vi "Stage and Sensor.vi"() -> ()   [LabVIEW 2025]
uses:
  \\chem-fs-prd-01\cyran_research/Users/Erykah F/Vertical Stage + Sensor/ThorLabs.MotionControl.KCube.PositionAlignerCLI.dll
  Vertical Stage + Sensor/ThorLabs.MotionControl.KCube.PositionAlignerCLI.dll
  Vertical Stage + Sensor/libximc.lvlib
  \\chem-fs-prd-01\cyran_research/Users/Erykah F/Vertical Stage + Sensor/Thorlabs.MotionControl.Controls.dll
  Vertical Stage + Sensor/Thorlabs.MotionControl.Controls.dll
panel:
  out "Y diff":dbl
  out "X diff":dbl
  out "Sum":dbl
  in  "KCubePositionAlignerControl":refnum<k24>(container)
  in  "Tab Control":T1(tab)
  in  "Controller 3":u16(ring) items=["xi-com:\\\\.\\COM4", "xi-com:\\\\.\\COM5", "xi-com:\\\\.\\COM6"]
  in  "Controller 2":u16(ring) items=["xi-com:\\\\.\\COM4", "xi-com:\\\\.\\COM5", "xi-com:\\\\.\\COM6"]
  in  "Controller 1":u16(ring) items=["xi-com:\\\\.\\COM4", "xi-com:\\\\.\\COM5", "xi-com:\\\\.\\COM6"]
  out "s/n 1":u32
  out "s/n 3":u32
  out "s/n 2":u32
  in  "KCube Serial  Number":string="69254064"
  in  "Move To Destination":bool
  in  "Move Relative":bool
  in  "Shift 1":i32
  in  "Shift 2":i32
  in  "Shift 3":i32
  in  "Destination 3":i32
  in  "Destination 2":i32
  in  "Destination 1":i32
  in  "Loop?":bool caption="Loop Shift?"
  in  "Shift Amount (Steps)":i32=1
  in  "Wait Time (s)":dbl=1.0
  in  "Exit":bool
  out "Cursor 3":dbl format="%#.2f"
  out "Cursor 2":dbl format="%#.2f"
  out "Cursor 1":dbl format="%#.2f"
  # "Position Status"
  # "\\_(-_ -)_/"
  # "Controller IDs"
  # "Serial Numbers"
  # "Disabled because we don't usually use this function"
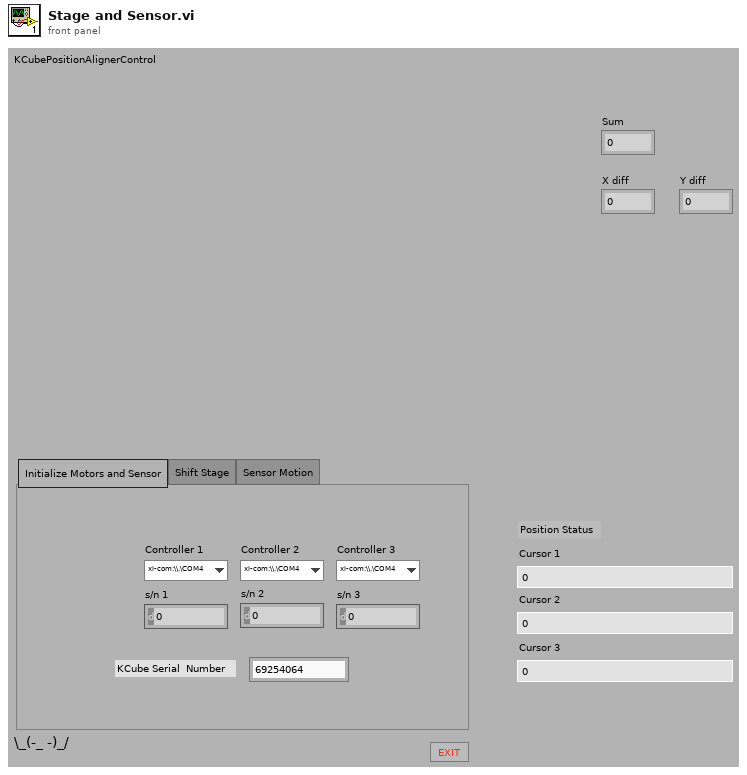
[diagram p1: front panel]
types:
  T1 = enum32{"Initialize Motors and Sensor", "Shift Stage", "Sensor Motion"}
  T2 = cluster{"Number of controllers":i32, "Controllers' names":string[], "variant":variant, "quit":bool, "IDs":i32[]}
  T3 = cluster{"KCubePositionAlignerControl":refnum<k24>, "Device":refnum<k24>, dbl, dbl, dbl, dbl}
  T4 = cluster{"MoveSts":u32, "MvCmdSts":u32, "PWRSts":u32, "EncSts":u32, "WindSts":u32, "CurPosition":i32, "uCurPosition":i32, "@dummy control@":i8, "@dummy control@":i8, "@dummy control@":i8, "@dummy control@":i8, "EncPosition":i64, "CurSpeed":i32, "uCurSpeed":i32, "Ipwr":i32, "Upwr":i32, "Iusb":i32, "Uusb":i32, "CurT":i32, "Flags":u32, "GPIOFlags":u32, "CmdBufFreeSpace":u32}
  T5 = cluster{"Shift 1":i32, "Shift 2":i32, "Shift 3":i32}
  T6 = cluster{"Destination 1":i32, "Destination 2":i32, "Destination 3":i32}
  T7 = cluster{"Shift Amount (Steps)":i32, "Shift Amount (Steps)":i32, "Shift Amount (Steps)":i32}
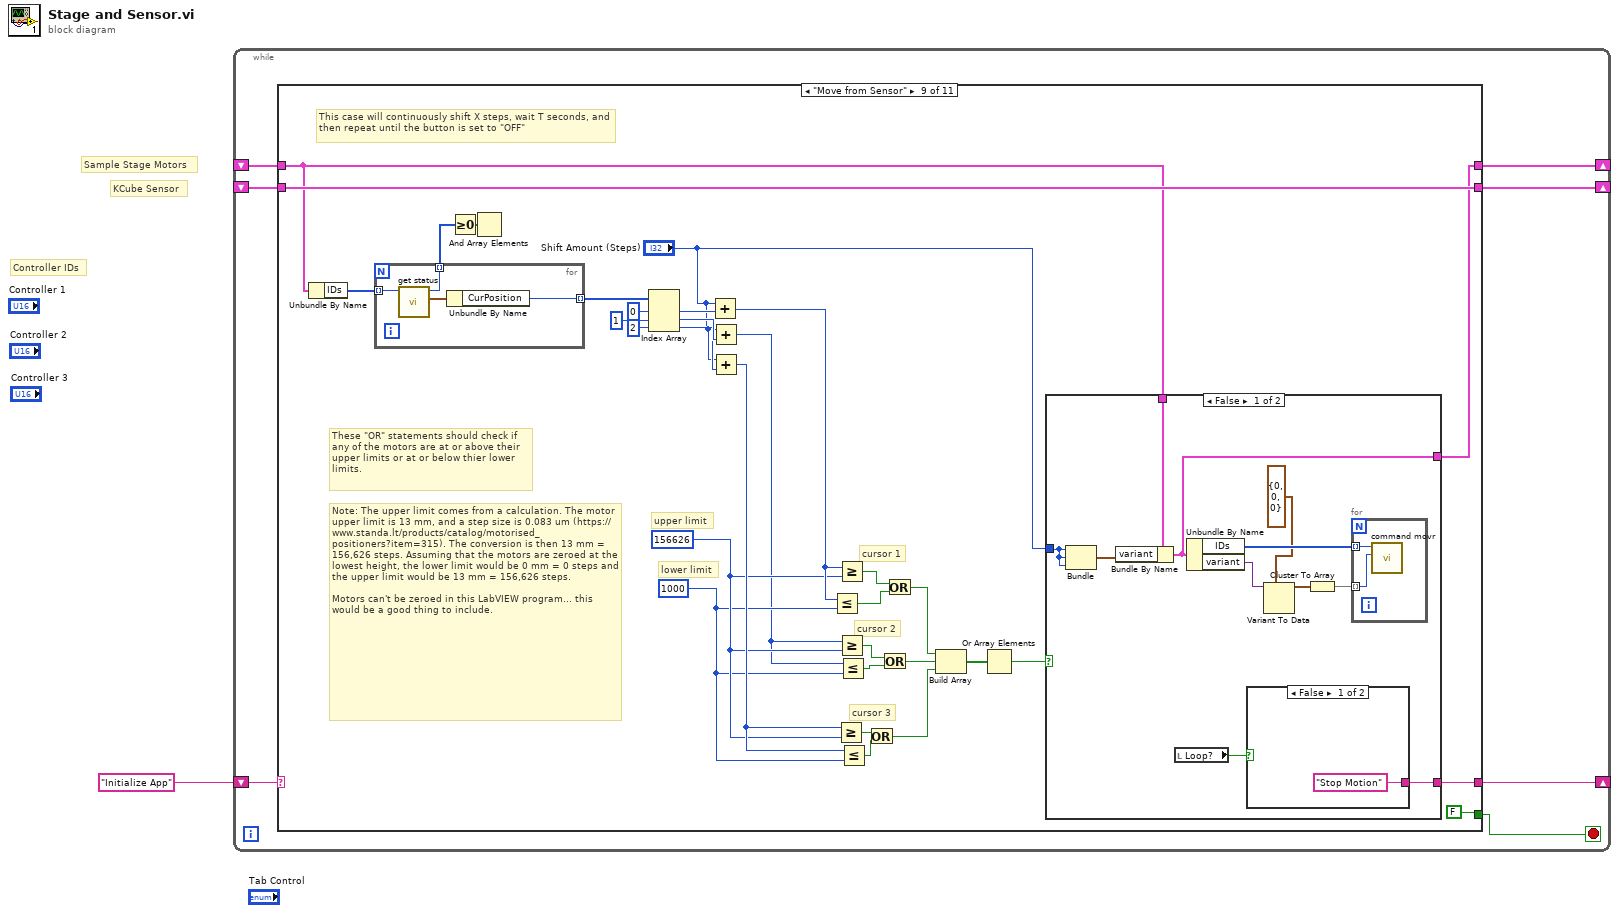
[diagram p0: block diagram]
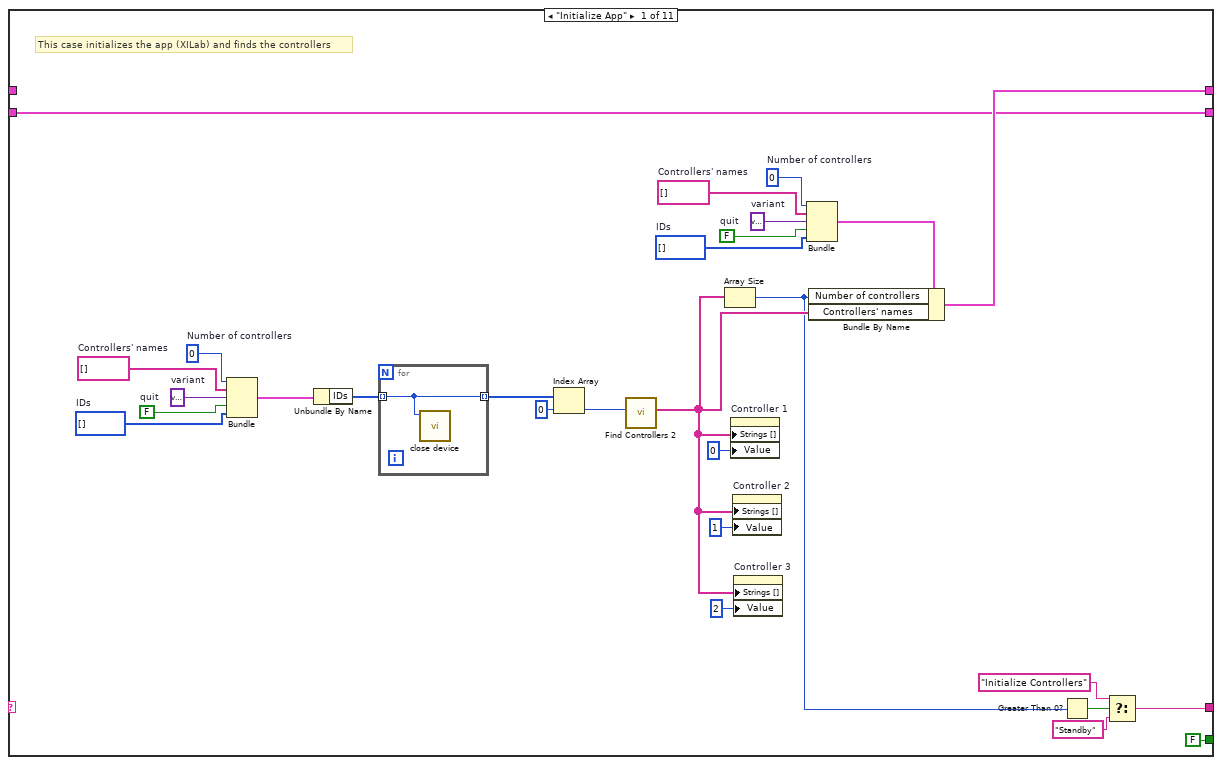
[diagram p2: hidden frame]
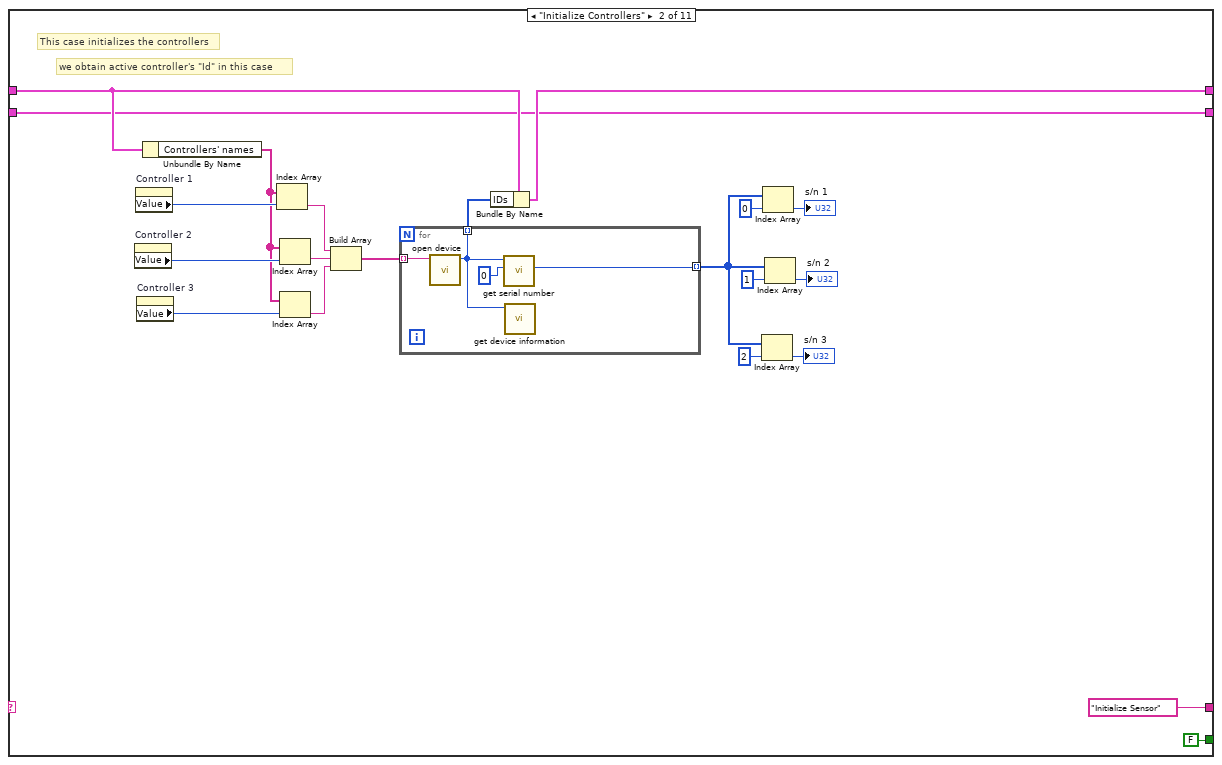
[diagram p3: hidden frame]
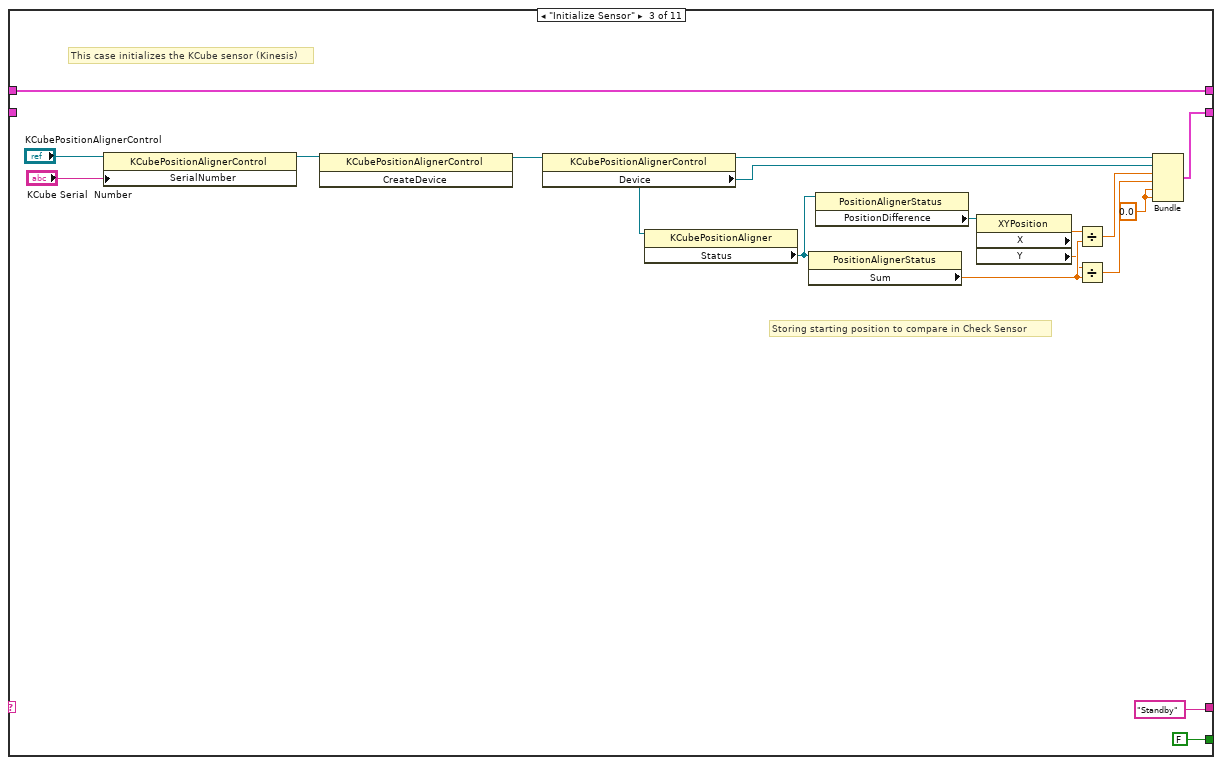
[diagram p4: hidden frame]
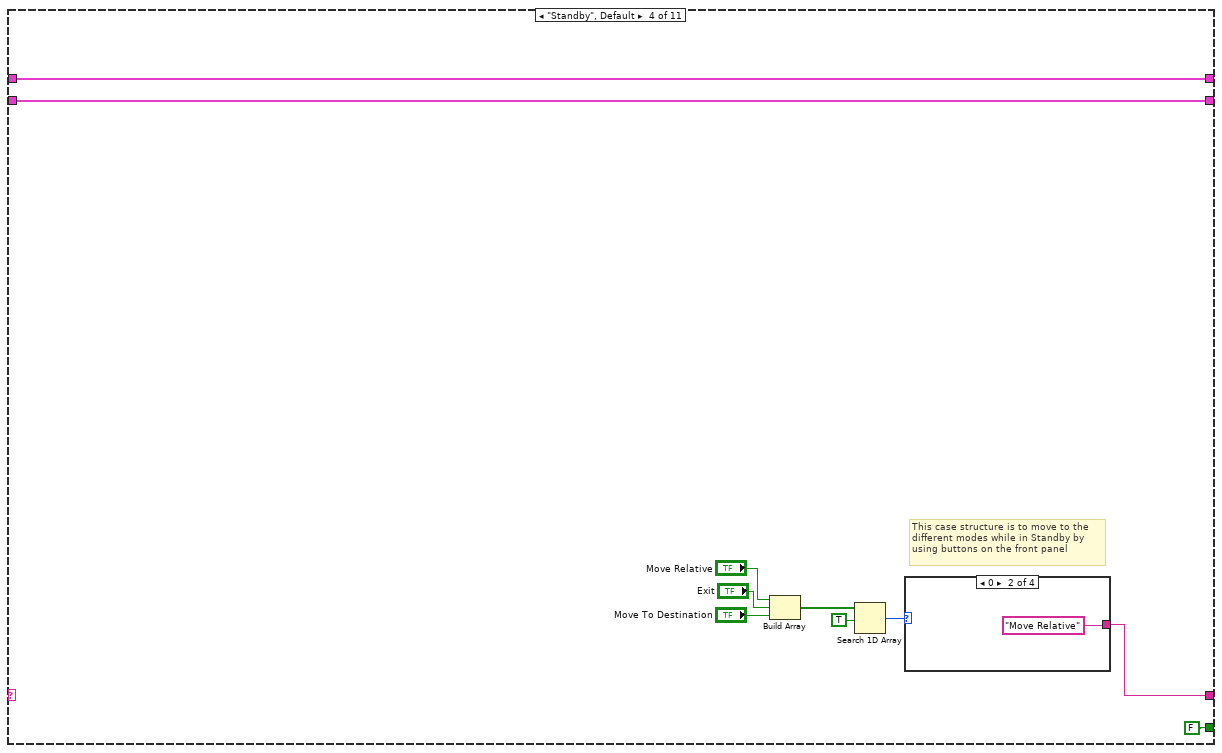
[diagram p5: hidden frame]
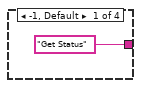
[diagram p6: hidden frame]
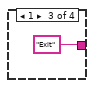
[diagram p7: hidden frame]
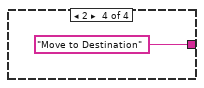
[diagram p8: hidden frame]
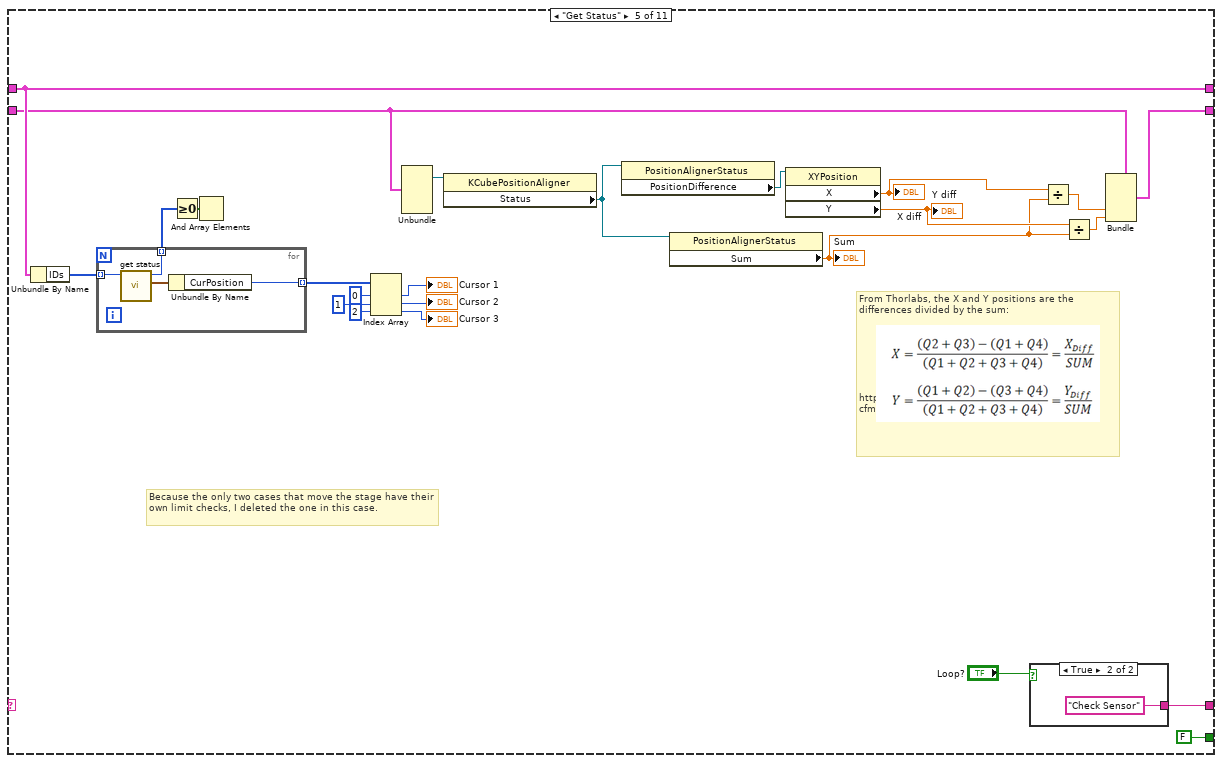
[diagram p9: hidden frame]
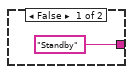
[diagram p10: hidden frame]
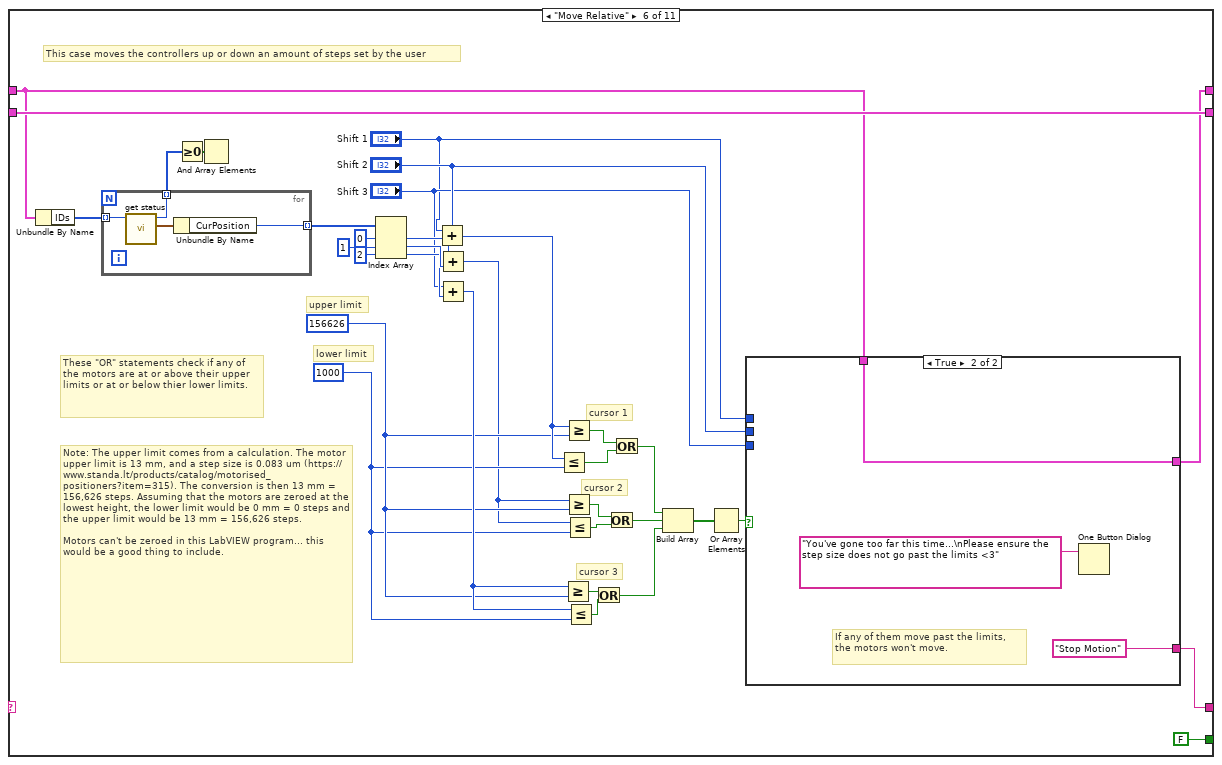
[diagram p11: hidden frame]
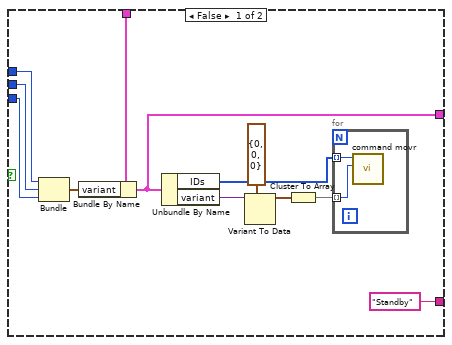
[diagram p12: hidden frame]
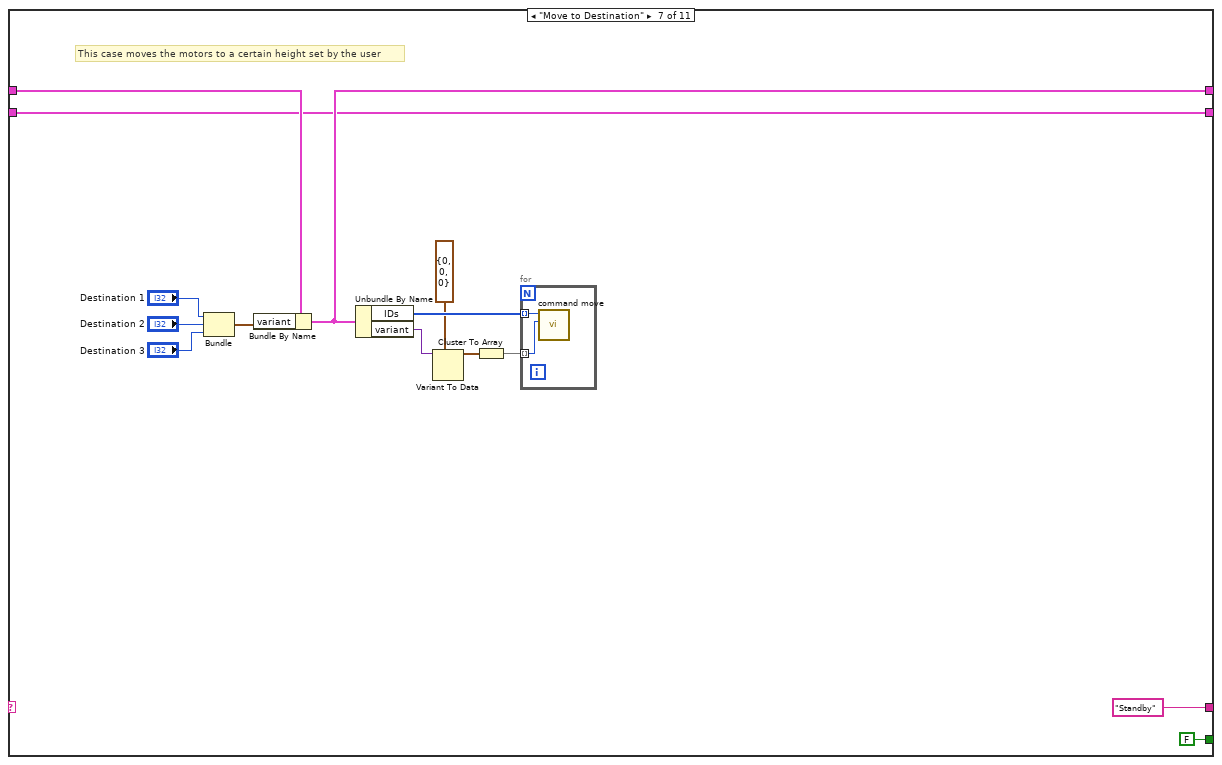
[diagram p13: hidden frame]
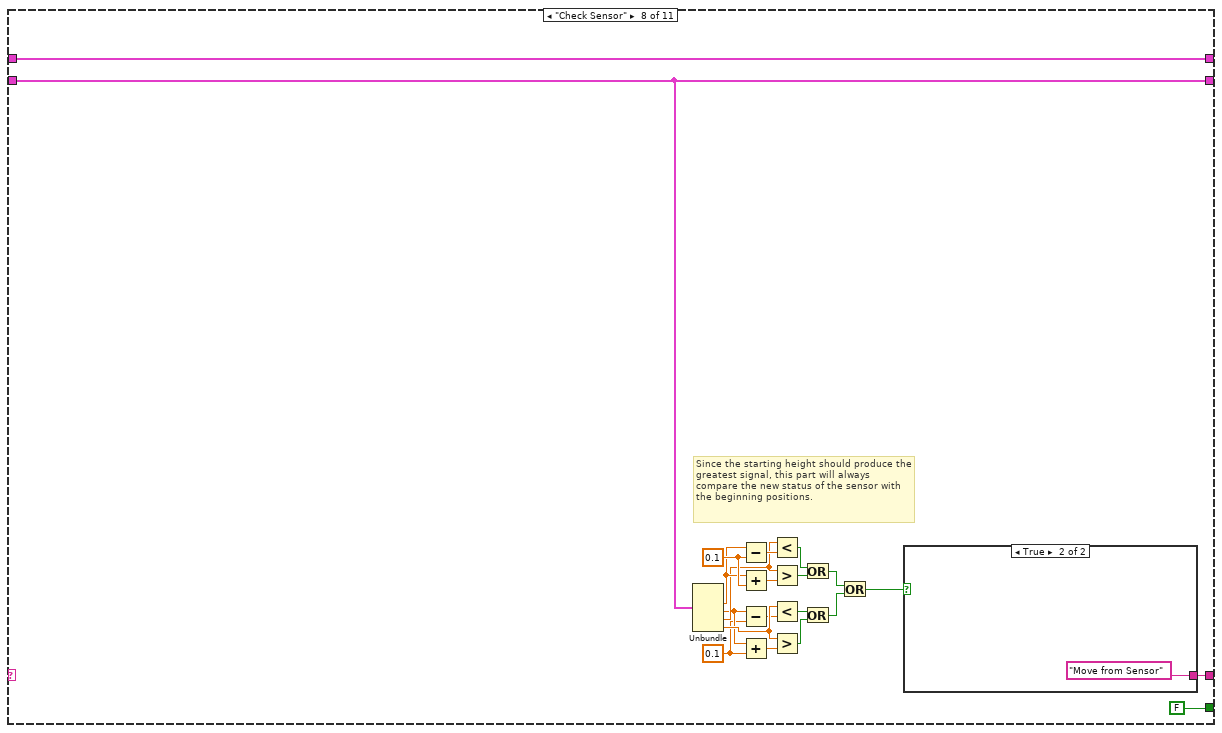
[diagram p14: hidden frame]
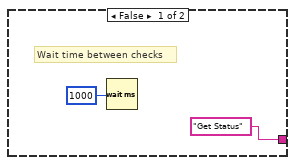
[diagram p15: hidden frame]
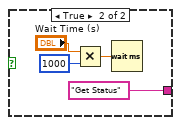
[diagram p16: hidden frame]
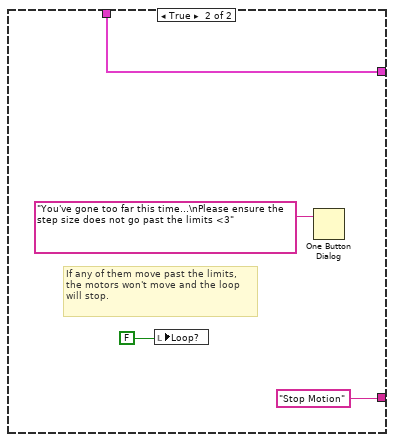
[diagram p17: hidden frame]
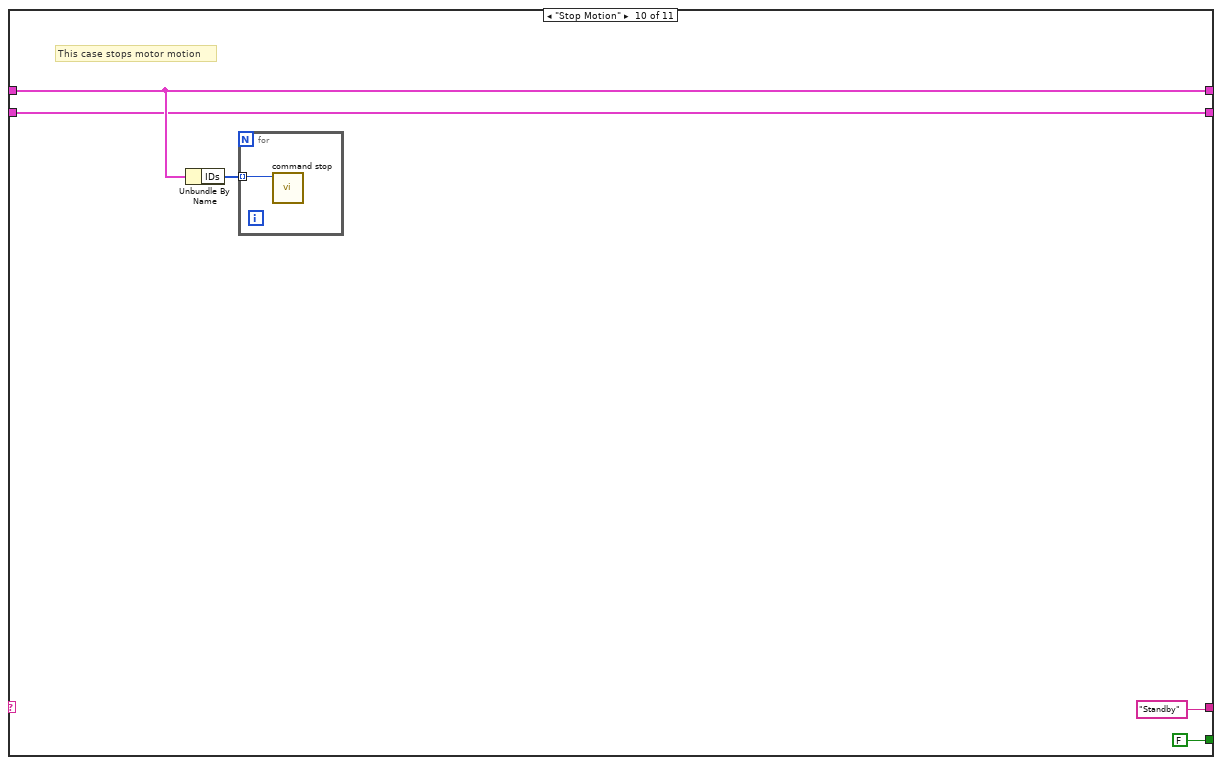
[diagram p18: hidden frame]
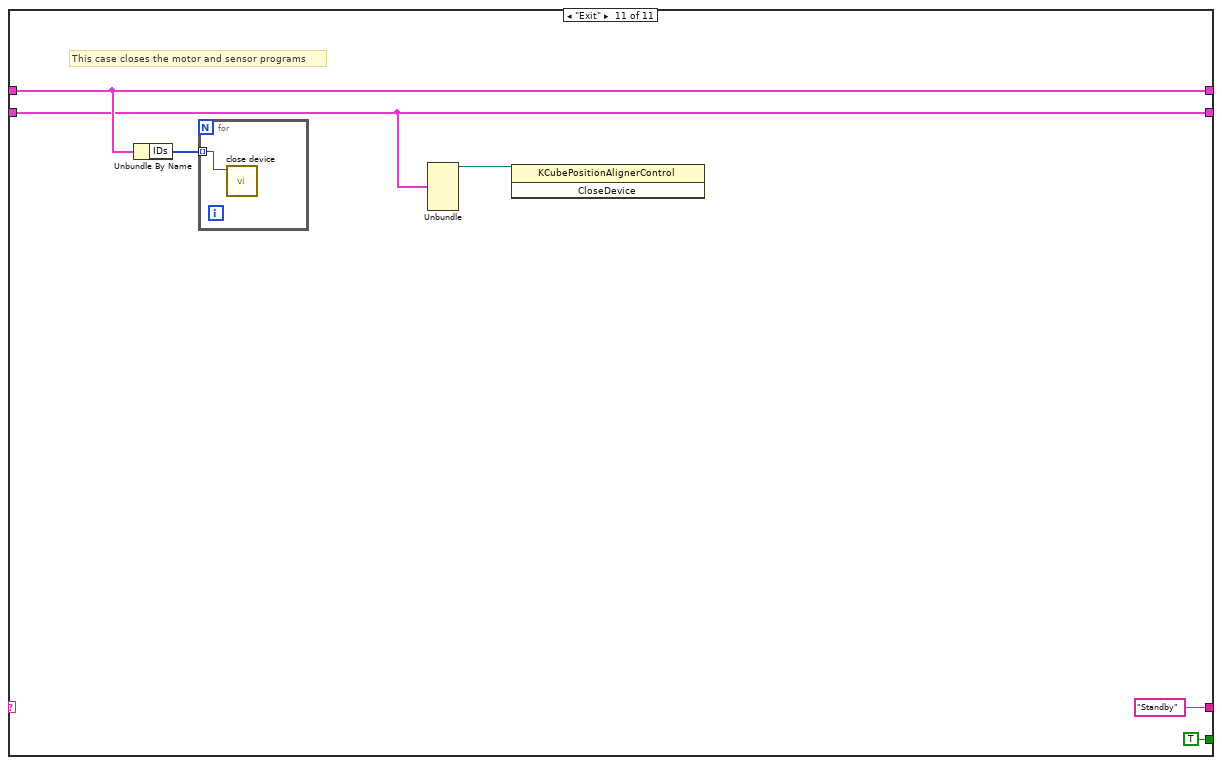
[diagram p19: hidden frame]
diagram:
  # "KCube Sensor"
  # "Sample Stage Motors"
  # "Controller IDs"
  n1 = while {
    shift-right: [w7] -> _
    shift-left: _ -> [w8]
    shift-right: [w6] -> _
    shift-left: "Initialize App" -> [w5]
    shift-right: [w3] -> _
    shift-left: _ -> [w2]
    stop <- w4 stop-if-true
    n2 = case shown="\"Move from Sensor\"" w5 {
      tunnel: [w30 w48 w79 w90 w111 w126 w182 w216 w221 w279 w287] -> w7
      tunnel: w8 -> [_ w49 w79 w90 w111 w127 w184 w216 w222 w279 w287]
      tunnel: [w11 "Initialize Sensor" "Standby" w84 w96 w139 "Standby" w214 w251 "Standby" "Standby"] -> w6
      tunnel: [FALSE ("quit") FALSE ("quit") FALSE FALSE ("quit") FALSE ("quit") FALSE ("quit") FALSE ("quit") FALSE FALSE FALSE TRUE ("quit")] -> w4
      tunnel: [w9 w38 w73 w82 w104 w158 w180 w213 w249 w278 w284] -> w3
      tunnel: w2 -> [w9 w38 _ w82 w103 w158 w180 w213 w249 w278 w284]
      frame "Initialize App" {
        w17 = i32[] []  # IDs
        w18 = FALSE  # quit
        w19 = variant  # variant
        w20 = string[] []  # Controllers' names
        w21 = 0  # Number of controllers
        w32 = i32[] []  # IDs
        w33 = FALSE  # quit
        w34 = variant  # variant
        w35 = string[] []  # Controllers' names
        w36 = 0  # Number of controllers
        # "This case initializes the app (XILab) and finds the controllers"
        n3 = Bundle("Number of controllers"=w21, "Controllers' names"=w20, "variant"=w19, "quit"=w18, "IDs"=w17) -> (w16:T2)  [unwired: 1 in]
        n4 = Unbundle By Name(w16) -> ("IDs"=w23:i32[])
        n5 = for {
          tunnel: w23 -> [w37] mode=indexing
          tunnel: [w37] -> w22 mode=indexing
          n6 = call "close device.vi"("id"=w37) -> ()  [unwired: 8 in, 3 out]
        }
        n7 = Index Array(array=w22, index=0) -> (element=w28:i32)
        n8 = call "Find Controllers 2.vi"("Numeric"=w28) -> ("Names"=w24:string[])  [unwired: 9 in, 1 out]
        n9 = Array Size(array=w24) -> (size(s)=w14:i32)
        n10 = property on="Controller 1" class="Ring (strict)"("Strings []"=w24, "Value"=0) -> ()  [unwired: 2 in, 2 out]
        n11 = property on="Controller 2" class="Ring (strict)"("Strings []"=w24, "Value"=1) -> ()  [unwired: 2 in, 2 out]
        n12 = property on="Controller 3" class="Ring (strict)"("Strings []"=w24, "Value"=2 ("Controller 3")) -> ()  [unwired: 2 in, 2 out]
        n13 = Bundle("Number of controllers"=w36, "Controllers' names"=w35, "variant"=w34, "quit"=w33, "IDs"=w32) -> (w31:T2)  [unwired: 1 in]
        n14 = Bundle By Name(cluster=w31, "Number of controllers"=w14, "Controllers' names"=w24) -> (w30:T2)
        n15 = Greater Than 0?(x=w14) -> (x > 0?=w15:bool)
        n16 = Select(t="Initialize Controllers", s=w15, f="Standby") -> (s? t:f=w11:string)
      }
      frame "Initialize Controllers" {
        # "we obtain active controller's \"Id\" in this case"
        # "This case initializes the controllers"
        n17 = property on="Controller 2" class="Ring (strict)"() -> ("Value"=w57:u16)  [unwired: 2 in, 2 out]
        n18 = property on="Controller 1" class="Ring (strict)"() -> ("Value"=w58:u16)  [unwired: 2 in, 2 out]
        n19 = property on="Controller 3" class="Ring (strict)"() -> ("Value"=w56:u16)  [unwired: 2 in, 2 out]
        n20 = Unbundle By Name(w49) -> ("Controllers' names"=w52:string[])
        n21 = Index Array(array=w52, index=w58) -> (element=w53:string)
        n22 = Index Array(array=w52, index=w57) -> (element=w54:string)
        n23 = Index Array(array=w52, index=w56) -> (element=w55:string)
        n24 = Build Array(w53, w54, w55) -> (w51:string[])
        n25 = for {
          tunnel: w51 -> [w62] mode=indexing
          tunnel: [w60] -> w50 mode=indexing
          tunnel: [w61] -> w41 mode=indexing
          n26 = call "open device.vi"("uri"=w62) -> ("function return"=w60:i32)  [unwired: 9 in, 1 out]
          n27 = call "get serial number.vi"("SerialNumber"=0, "id"=w60) -> ("SerialNumber out"=w61:u32)  [unwired: 7 in, 2 out]
          n28 = call "get device information.vi"("id"=w60) -> ()  [unwired: 8 in, 3 out]
        }
        n29 = Bundle By Name(cluster=w49, "IDs"=w50) -> (w48:T2)
        n30 = Index Array(array=w41, index=u32 2 ("serial")) -> (element=→"s/n 3":u32)
        n31 = Index Array(array=w41, index=u32 0 ("serial")) -> (element=→"s/n 1":u32)
        n32 = Index Array(array=w41, index=u32 1 ("serial")) -> (element=→"s/n 2":u32)
      }
      frame "Initialize Sensor" {
        w71 = 0.0
        # "Storing starting position to compare in Check Sensor"
        # "This case initializes the KCube sensor (Kinesis)"
        n33 = property class="KCubePositionAlignerControl"(reference="KCubePositionAlignerControl", "SerialNumber"="KCube Serial  Number") -> (reference out=w77:refnum<k24>)  [unwired: 1 in, 1 out]
        n34 = invoke class="KCubePositionAlignerControl" method="CreateDevice"(reference=w77) -> (reference out=w76:refnum<k24>)  [unwired: 2 in, 2 out]
        n35 = property class="KCubePositionAlignerControl"(reference=w76) -> (reference out=w74:refnum<k24>, "Device"=w68:refnum<k24>)  [unwired: 1 in, 1 out]
        n36 = property class="KCubePositionAligner"(reference=w68) -> ("Status"=w69:refnum<k24>)  [unwired: 1 in, 2 out]
        n37 = property class="PositionAlignerStatus"(reference=w69) -> ("Sum"=w67:dbl)  [unwired: 1 in, 2 out]
        n38 = property class="PositionAlignerStatus"(reference=w69) -> ("PositionDifference"=w70:refnum<k24>)  [unwired: 1 in, 2 out]
        n39 = property class="XYPosition"(reference=w70) -> ("X"=w66:dbl, "Y"=w65:dbl)  [unwired: 1 in, 2 out]
        n40 = Divide(x=w66, y=w67) -> (x/y=w64:dbl)
        n41 = Divide(x=w65, y=w67) -> (x/y=w63:dbl)
        n42 = Bundle("KCubePositionAlignerControl"=w74, "Device"=w68, w64, w63, w71, w71) -> (w73:T3)  [unwired: 1 in]
      }
      frame "Standby", Default {
        # "This case structure is to move to the different modes while in Standby by using buttons on the front panel"
        n43 = Build Array("Move Relative", "Exit", "Move To Destination") -> (w87:bool[])
        n44 = Search 1D Array(1D array=w87, element=TRUE) -> (index of element=w85:i32)  [unwired: 1 in]
        n45 = case shown="0" w85 {
          tunnel: ["Get Status" "Move Relative" "Exit" "Move to Destination"] -> w84
          frame -1, Default {
          }
          frame 0 {
          }
          frame 1 {
          }
          frame 2 {
          }
        }
      }
      frame "Get Status" {
        # "Because the only two cases that move the stage have their own limit checks, I deleted the one in this case."
        # "From Thorlabs, the X and Y positions are the differences divided by the sum: \n\n\n\n\n\n\n\nhttps://www.thorlabs.com/newgrouppage9.cfm?objectgroup_ID=4400"
        n46 = Unbundle By Name(w111) -> ("IDs"=w118:i32[])
        n47 = for {
          tunnel: [w124] -> w116 mode=indexing
          tunnel: w118 -> [w123] mode=indexing
          tunnel: [w122] -> w117 mode=indexing
          n48 = call "get status.vi"("id"=w123) -> ("status out"=w121:T4, "function return"=w122:i32)  [unwired: 8 in, 1 out]
          n49 = Unbundle By Name(w121) -> ("CurPosition"=w124:i32)
        }
        n50 = Greater Or Equal To 0?(x=w117) -> (x >= 0?=w112:bool[])
        n51 = And Array Elements(Boolean array=w112) -> ()  [unwired: 1 out]
        n52 = Index Array(array=w116, index #1=0 ("index"), index #2=1 ("index"), index #3=2 ("index")) -> (element #1=→"Cursor 1":i32, element #2=→"Cursor 2":i32, element #3=→"Cursor 3":i32)
        n53 = Unbundle(w103) -> ("Device"=w106:refnum<k24>)  [unwired: 5 out]
        n54 = property class="KCubePositionAligner"(reference=w106) -> ("Status"=w105:refnum<k24>)  [unwired: 1 in, 2 out]
        n55 = property class="PositionAlignerStatus"(reference=w105) -> ("PositionDifference"=w107:refnum<k24>)  [unwired: 1 in, 2 out]
        n56 = property class="PositionAlignerStatus"(reference=w105) -> ("Sum"=w100:dbl)  [unwired: 1 in, 2 out]
        "Sum" <- w100
        n57 = property class="XYPosition"(reference=w107) -> ("X"=w102:dbl, "Y"=w101:dbl)  [unwired: 1 in, 2 out]
        "X diff" <- w102
        "Y diff" <- w101
        n58 = case shown="True" "Loop?" {
          tunnel: ["Standby" "Check Sensor"] -> w96
          frame False {
          }
          frame True {
          }
        }
        n59 = Divide(x=w102, y=w100) -> (x/y=w98:dbl)
        n60 = Divide(x=w101, y=w100) -> (x/y=w99:dbl)
        n61 = Bundle(cluster=w103, w98, w99) -> (w104:T3)  [unwired: 4 in]
      }
      frame "Move Relative" {
        w132 = 1000
        w133 = 156626
        # "cursor 3"
        # "cursor 2"
        # "cursor 1"
        # "lower limit"
        # "upper limit"
        # "Note: The upper limit comes from a calculation. The motor upper limit is 13 mm, and a step size is 0.083 um (https://www.standa.lt/products/catalog/motorised_positioners?item=315). The conversion is then 13 mm = 156,626 steps. Assuming that the motors are zeroed at the lowest height, the lower limit would be 0 mm = 0 steps and the upper limit would be 13 mm = 156,626 steps.\n\nMotors can't be zeroed in this LabVIEW program... this would be a good thing to include."
        # "These \"OR\" statements check if any of the motors are at or above their upper limits or at or below thier lower limits."
        # "This case moves the controllers up or down an amount of steps set by the user"
        n62 = Unbundle By Name(w127) -> ("IDs"=w157:i32[])
        n63 = for {
          tunnel: [w179] -> w155 mode=indexing
          tunnel: w157 -> [w178] mode=indexing
          tunnel: [w177] -> w156 mode=indexing
          n64 = call "get status.vi"("id"=w178) -> ("status out"=w176:T4, "function return"=w177:i32)  [unwired: 8 in, 1 out]
          n65 = Unbundle By Name(w176) -> ("CurPosition"=w179:i32)
        }
        n66 = Greater Or Equal To 0?(x=w156) -> (x >= 0?=w151:bool[])
        n67 = And Array Elements(Boolean array=w151) -> ()  [unwired: 1 out]
        n68 = Index Array(array=w155, index #1=0 ("index"), index #2=1 ("index"), index #3=2 ("index")) -> (element #1=w138:i32, element #2=w137:i32, element #3=w136:i32)
        n69 = Add(x="Shift 1", y=w138) -> (x+y=w135:i32)
        n70 = Add(x="Shift 2", y=w137) -> (x+y=w131:i32)
        n71 = Add(x="Shift 3", y=w136) -> (x+y=w134:i32)
        n72 = Less Or Equal?(x=w135, y=w132) -> (x <= y?=w149:bool)
        n73 = Greater Or Equal?(x=w134, y=w133) -> (x >= y?=w146:bool)
        n74 = Greater Or Equal?(x=w135, y=w133) -> (x >= y?=w150:bool)
        n75 = Greater Or Equal?(x=w131, y=w133) -> (x >= y?=w148:bool)
        n76 = Less Or Equal?(x=w131, y=w132) -> (x <= y?=w147:bool)
        n77 = Less Or Equal?(x=w134, y=w132) -> (x <= y?=w145:bool)
        n78 = Or(x=w146, y=w145) -> (x .or. y?=w142:bool)
        n79 = Or(x=w148, y=w147) -> (x .or. y?=w143:bool)
        n80 = Or(x=w150, y=w149) -> (x .or. y?=w144:bool)
        n81 = Build Array(w144, w143, w142) -> (w141:bool[])
        n82 = Or Array Elements(Boolean array=w141) -> (logical OR=w140:bool)
        n83 = case shown="True" w140 {
          tunnel: ["Standby" "Stop Motion"] -> w139
          tunnel: "Shift 1" -> [w169 _]
          tunnel: "Shift 2" -> [w168 _]
          tunnel: "Shift 3" -> [w167 _]
          tunnel: w127 -> [w166 w173]
          tunnel: [w164 w173] -> w126
          frame False {
            n84 = Bundle("Shift 1"=w169, "Shift 2"=w168, "Shift 3"=w167) -> (w165:T5)  [unwired: 1 in]
            n85 = Bundle By Name(cluster=w166, "variant"=w165) -> (w164:T2)
            n86 = Unbundle By Name(w164) -> ("IDs"=w159:i32[], "variant"=w161:variant)
            n87 = Variant To Data(type=cluster{u32, u32, u32} {0, 0, 0}, Variant=w161) -> (data=w162:cluster{u32, u32, u32})  [unwired: 1 in, 1 out]
            n88 = Cluster To Array(cluster=w162) -> (array=w163:u32[])
            n89 = for {
              tunnel: w163 -> [w171] mode=indexing
              tunnel: w159 -> [w172] mode=indexing
              n90 = call "command movr.vi"("DeltaPosition"=w171, "id"=w172) -> ()  [unwired: 8 in, 2 out]
            }
          }
          frame True {
            # "If any of them move past the limits, the motors won't move."
            n91 = One Button Dialog(message="You've gone too far this time...\nPlease ensure the step size does not go past the limits <3") -> ()  [unwired: 1 in, 1 out]
          }
        }
      }
      frame "Move to Destination" {
        # "This case moves the motors to a certain height set by the user"
        n92 = Bundle("Destination 1"="Destination 1", "Destination 2"="Destination 2", "Destination 3"="Destination 3") -> (w193:T6)  [unwired: 1 in]
        n93 = Bundle By Name(cluster=w184, "variant"=w193) -> (w182:T2)
        n94 = Unbundle By Name(w182) -> ("IDs"=w188:i32[], "variant"=w185:variant)
        n95 = Variant To Data(type=cluster{u32, u32, u32} {0, 0, 0}, Variant=w185) -> (data=w189:cluster{u32, u32, u32})  [unwired: 1 in, 1 out]
        n96 = Cluster To Array(cluster=w189) -> (array=w186:u32[])
        n97 = for {
          tunnel: w186 -> [w194] mode=indexing
          tunnel: w188 -> [w195] mode=indexing
          n98 = call "command move.vi"("Position"=w194, "id"=w195) -> ()  [unwired: 8 in, 2 out]
        }
      }
      frame "Check Sensor" {
        w198 = 0.1
        w204 = 0.1
        # "Since the starting height should produce the greatest signal, this part will always compare the new status of the sensor with the beginning positions."
        n99 = Unbundle(w213) -> (w203:dbl, w199:dbl, w200:dbl, w211:dbl)  [unwired: 2 out]
        n100 = Subtract(x=w203, y=w204) -> (x-y=w201:dbl)
        n101 = Add(x=w203, y=w204) -> (x+y=w202:dbl)
        n102 = Subtract(x=w199, y=w198) -> (x-y=w196:dbl)
        n103 = Add(x=w199, y=w198) -> (x+y=w197:dbl)
        n104 = Less?(x=w200, y=w201) -> (x < y?=w210:bool)
        n105 = Greater?(x=w200, y=w202) -> (0:w209:bool)
        n106 = Less?(x=w211, y=w196) -> (x < y?=w208:bool)
        n107 = Greater?(x=w211, y=w197) -> (0:w207:bool)
        n108 = Or(x=w210, y=w209) -> (x .or. y?=w205:bool)
        n109 = Or(x=w208, y=w207) -> (x .or. y?=w206:bool)
        n110 = Or(x=w205, y=w206) -> (x .or. y?=w212:bool)
        n111 = case shown="True" w212 {
          tunnel: ["Get Status" "Move from Sensor"] -> w214
          frame False {
            # "Wait time between checks"
            n112 = Wait (ms)(milliseconds to wait=1000) -> ()  [unwired: 1 out]
          }
          frame True {
          }
        }
      }
      frame "Move from Sensor" {
        w225 = 1000
        w226 = 156626
        # "Note: The upper limit comes from a calculation. The motor upper limit is 13 mm, and a step size is 0.083 um (https://www.standa.lt/products/catalog/motorised_positioners?item=315). The conversion is then 13 mm = 156,626 steps. Assuming that the motors are zeroed at the lowest height, the lower limit would be 0 mm = 0 steps and the upper limit would be 13 mm = 156,626 steps.\n\nMotors can't be zeroed in this LabVIEW program... this would be a good thing to include."
        # "These \"OR\" statements should check if any of the motors are at or above their upper limits or at or below thier lower limits."
        # "cursor 3"
        # "cursor 2"
        # "cursor 1"
        # "lower limit"
        # "upper limit"
        # "This case will continuously shift X steps, wait T seconds, and then repeat until the button is set to \"OFF\""
        n113 = Unbundle By Name(w222) -> ("IDs"=w248:i32[])
        n114 = for {
          tunnel: [w277] -> w246 mode=indexing
          tunnel: w248 -> [w276] mode=indexing
          tunnel: [w275] -> w247 mode=indexing
          n115 = call "get status.vi"("id"=w276) -> ("status out"=w274:T4, "function return"=w275:i32)  [unwired: 8 in, 1 out]
          n116 = Unbundle By Name(w274) -> ("CurPosition"=w277:i32)
        }
        n117 = Greater Or Equal To 0?(x=w247) -> (x >= 0?=w242:bool[])
        n118 = And Array Elements(Boolean array=w242) -> ()  [unwired: 1 out]
        n119 = Index Array(array=w246, index #1=0 ("index"), index #2=1 ("index"), index #3=2 ("index")) -> (element #1=w231:i32, element #2=w230:i32, element #3=w229:i32)
        n120 = Add(x="Shift Amount (Steps)", y=w231) -> (x+y=w228:i32)
        n121 = Add(x="Shift Amount (Steps)", y=w230) -> (x+y=w224:i32)
        n122 = Add(x="Shift Amount (Steps)", y=w229) -> (x+y=w227:i32)
        n123 = Less Or Equal?(x=w228, y=w225) -> (x <= y?=w240:bool)
        n124 = Greater Or Equal?(x=w227, y=w226) -> (x >= y?=w237:bool)
        n125 = Greater Or Equal?(x=w228, y=w226) -> (x >= y?=w241:bool)
        n126 = Greater Or Equal?(x=w224, y=w226) -> (x >= y?=w239:bool)
        n127 = Less Or Equal?(x=w224, y=w225) -> (x <= y?=w238:bool)
        n128 = Less Or Equal?(x=w227, y=w225) -> (x <= y?=w236:bool)
        n129 = Or(x=w237, y=w236) -> (x .or. y?=w233:bool)
        n130 = Or(x=w239, y=w238) -> (x .or. y?=w234:bool)
        n131 = Or(x=w241, y=w240) -> (x .or. y?=w235:bool)
        n132 = Build Array(w235, w234, w233) -> (w232:bool[])
        n133 = Or Array Elements(Boolean array=w232) -> (logical OR=w220:bool)
        n134 = case shown="False" w220 {
          tunnel: [w262 "Stop Motion"] -> w251
          tunnel: "Shift Amount (Steps)" -> [w252 _]
          tunnel: w222 -> [w254 w273]
          tunnel: [w253 w273] -> w221
          frame False {
            n135 = Bundle("Shift Amount (Steps)"=w252, "Shift Amount (Steps)"=w252, "Shift Amount (Steps)"=w252) -> (w256:T7)  [unwired: 1 in]
            n136 = Bundle By Name(cluster=w254, "variant"=w256) -> (w253:T2)
            n137 = local read "Loop?"() -> (w261:bool)
            n138 = Unbundle By Name(w253) -> ("IDs"=w258:i32[], "variant"=w260:variant)
            n139 = case shown="False" w261 {
              tunnel: ["Stop Motion" "Get Status"] -> w262
              frame False {
              }
              frame True {
                n140 = Multiply(x="Wait Time (s)", y=1000) -> (x*y=w267:dbl)
                n141 = Wait (ms)(milliseconds to wait=w267) -> ()  [unwired: 1 out]
              }
            }
            n142 = Variant To Data(type=cluster{u32, u32, u32} {0, 0, 0}, Variant=w260) -> (data=w257:cluster{u32, u32, u32})  [unwired: 1 in, 1 out]
            n143 = Cluster To Array(cluster=w257) -> (array=w259:u32[])
            n144 = for {
              tunnel: w259 -> [w263] mode=indexing
              tunnel: w258 -> [w264] mode=indexing
              n145 = call "command movr.vi"("DeltaPosition"=w263, "id"=w264) -> ()  [unwired: 8 in, 2 out]
            }
          }
          frame True {
            # "If any of them move past the limits, the motors won't move and the loop will stop."
            n146 = local write "Loop?"(FALSE) -> ()
            n147 = One Button Dialog(message="You've gone too far this time...\nPlease ensure the step size does not go past the limits <3") -> ()  [unwired: 1 in, 1 out]
          }
        }
      }
      frame "Stop Motion" {
        # "This case stops motor motion"
        n148 = Unbundle By Name(w279) -> ("IDs"=w280:i32[])
        n149 = for {
          tunnel: w280 -> [w283] mode=indexing
          n150 = call "command stop.vi"("id"=w283) -> ()  [unwired: 9 in, 2 out]
        }
      }
      frame "Exit" {
        # "This case closes the motor and sensor programs"
        n151 = Unbundle By Name(w287) -> ("IDs"=w289:i32[])
        n152 = for {
          tunnel: w289 -> [w290] mode=indexing
          n153 = call "close device.vi"("id"=w290) -> ()  [unwired: 8 in, 3 out]
        }
        n154 = Unbundle(w284) -> ("KCubePositionAlignerControl"=w285:refnum<k24>)  [unwired: 5 out]
        n155 = invoke class="KCubePositionAlignerControl" method="CloseDevice"(reference=w285) -> ()  [unwired: 2 in, 3 out]
      }
    }
  }
